vi "testbuffer.vi"(1 "Temp Config in":cluster{"timeout":dbl, "timeout 2":dbl}, 2 "command":string) -> (0 "Temp Config out":cluster{"timeout":dbl, "timeout 2":dbl})   [LabVIEW 2010]
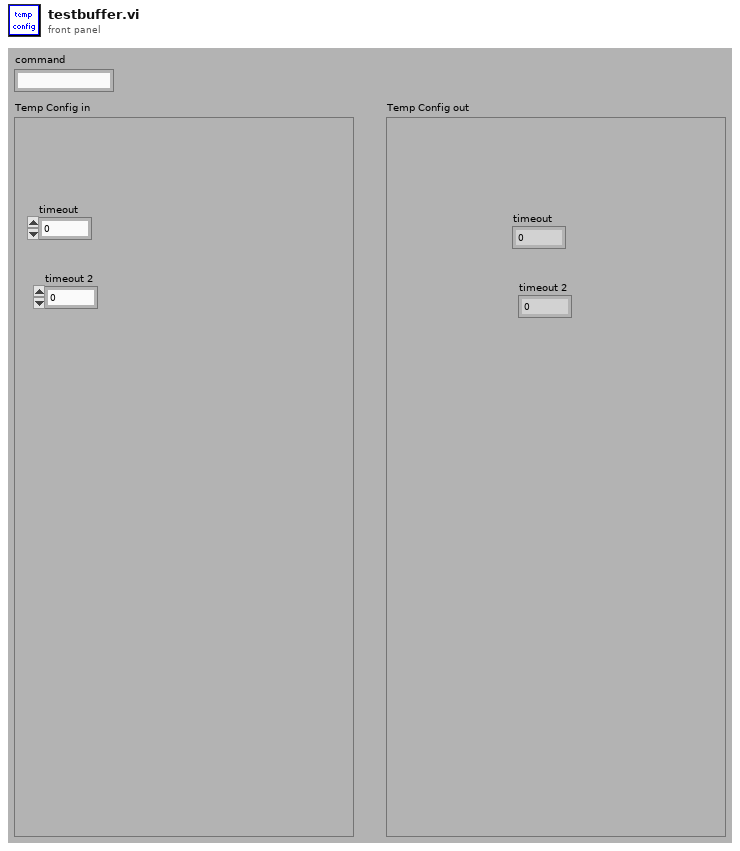
[diagram p1: front panel]
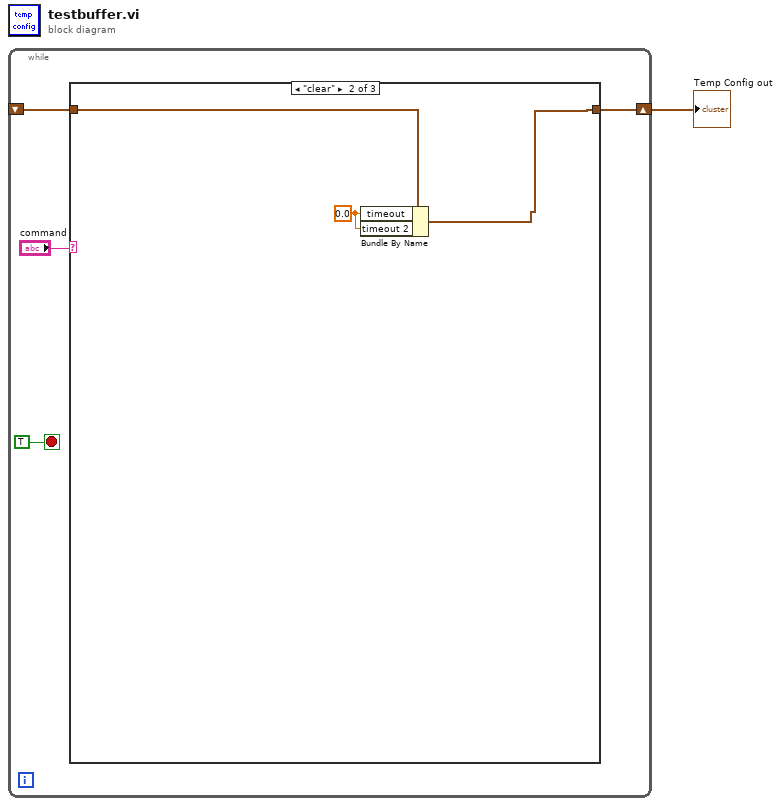
[diagram p0: block diagram]
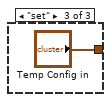
[diagram p3: hidden frame]
diagram:
  n1 = while {
    shift-right: [w3] -> w1
    shift-left: _ -> [w2]
    stop <- TRUE stop-if-true
    n2 = case shown="\"clear\"" "command" {
      tunnel: [w6 w8 "Temp Config in"] -> w3
      tunnel: w2 -> [w6 w9 _]
      frame "get", Default {
      }
      frame "clear" {
        w7 = 0.0 ("timeout")
        n3 = Bundle By Name(cluster=w9, "timeout"=w7, "timeout 2"=w7) -> (w8:cluster{"timeout":dbl, "timeout 2":dbl})
      }
      frame "set" {
      }
    }
  }
  "Temp Config out" <- w1
